vi "S2C_PCIe1762H_Proc_Globals.vi"() -> ()   [LabVIEW 2024]
panel:
  in  "Module":i32
  out "1762-Refs":string[][](array[string])
  in  "1762-VI":refnum<vi>
  in  "Device":string="DemoDevice"
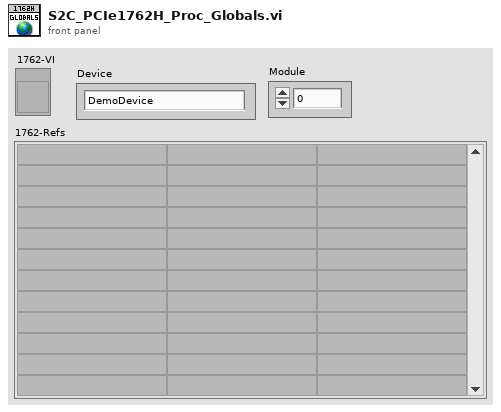
[diagram p1: front panel]
diagram:
